vi "Read DIP Switches.vi"() -> ()   [LabVIEW 2016]
uses:
  Source/GE 5565PIORC/Controls/S1 Switch.ctl
  Source/GE 5565PIORC/GE 5565PIORC Old.lvclass/GE 5565PIORC Old.ctl
  Source/GE 5565PIORC/VIs/Registers/Local Configuration.LAS1RR.Address Range.Get.vi
  Source/GE 5565PIORC/VIs/Registers/RFM Control and Status.LCSR1.Redundant Mode Enable.Get.vi
  Source/GE 5565PIORC/VIs/Registers/RFM Control and Status.LCSR1.Rogue Master 0 Enabled.Get.vi
  Source/GE 5565PIORC/VIs/Registers/RFM Control and Status.LCSR1.Rogue Master 1 Enabled.Get.vi
  Source/GE 5565PIORC/VIs/Registers/RFM Control and Status.LCSR1.Window 1.Get.vi
  Source/GE 5565PIORC/VIs/Registers/RFM Control and Status.LCSR1.Window 0.Get.vi
  Source/GE 5565PIORC/VIs/Registers/RFM Control and Status.LCSR1.Delay TX from PCI Write.Get.vi
  Source/GE 5565PIORC/VIs/Registers/Local Configuration.Get Register Offset.vi
  Source/GE 5565PIORC/VIs/Binary Operations/Get Bits.vi
  Source/GE 5565PIORC/VIs/Binary Operations/Get Bits U32.vi
  Source/GE 5565PIORC/VIs/Registers/RFM Control and Status.Get Register Offset.vi
  Source/GE 5565PIORC/GE 5565PIORC Old.lvclass
panel:
  out "S1 Switch":T1
  in  "VISA resource name":refnum<visa-resource-name>
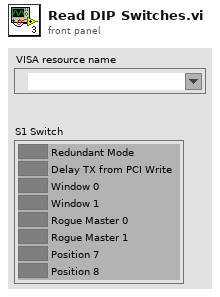
[diagram p1: front panel]
types:
  T1 = typedef "GE 5565PIORC Old.lvclass/S1 Switch.ctl" = cluster{"Redundant Mode":bool, "Delay TX from PCI Write":bool, "Window 0":bool, "Window 1":bool, "Rogue Master 0":bool, "Rogue Master 1":bool, "Position 7":bool, "Position 8":bool}
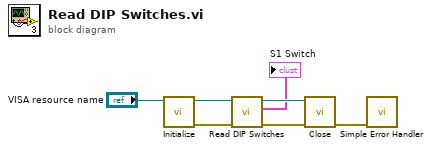
[diagram p0: block diagram]
diagram:
  n1 = call "Initialize.vi"("VISA resource name"="VISA resource name") -> ("error out"=w6:errorcluster, "GE 5565PIORC"=w7:refnum<class "GE 5565PIORC Old.lvclass">)  [unwired: 9 in]
  n2 = call "Read DIP Switches.vi"("error in (no error)"=w6, "GE 5565PIORC in"=w7) -> ("error out"=w3:errorcluster, "S1"=→"S1 Switch":T1, "GE 5565PIORC out"=w4:refnum<class "GE 5565PIORC Old.lvclass">)  [unwired: 7 in]
  n3 = call "Close.vi"("error in (no error)"=w3, "GE 5565PIORC in"=w4) -> ("error out"=w1:errorcluster)  [unwired: 8 in, 1 out]
  n4 = call <vilib>:"Simple Error Handler.vi"("error in (no error)"=w1) -> ()  [unwired: 4 in, 5 out]
